vi "montecarlo bpsk.vi"() -> ()   [LabVIEW 2014]
uses:
  <vilib>/Analysis/NI_AALBase.lvlib
panel:
  out "XY Graph":cluster{"Y":dbl[], "Y":dbl[]}[](graph)
  out "Waveform Chart 2":dbl[][](graph)
  out "Waveform Chart":i32[](graph)
  in  "Numeric 5":i32
  in  "Numeric 4":i32
  in  "Numeric 3":i32
  in  "Numeric 2":i32
  in  "Numeric":i32
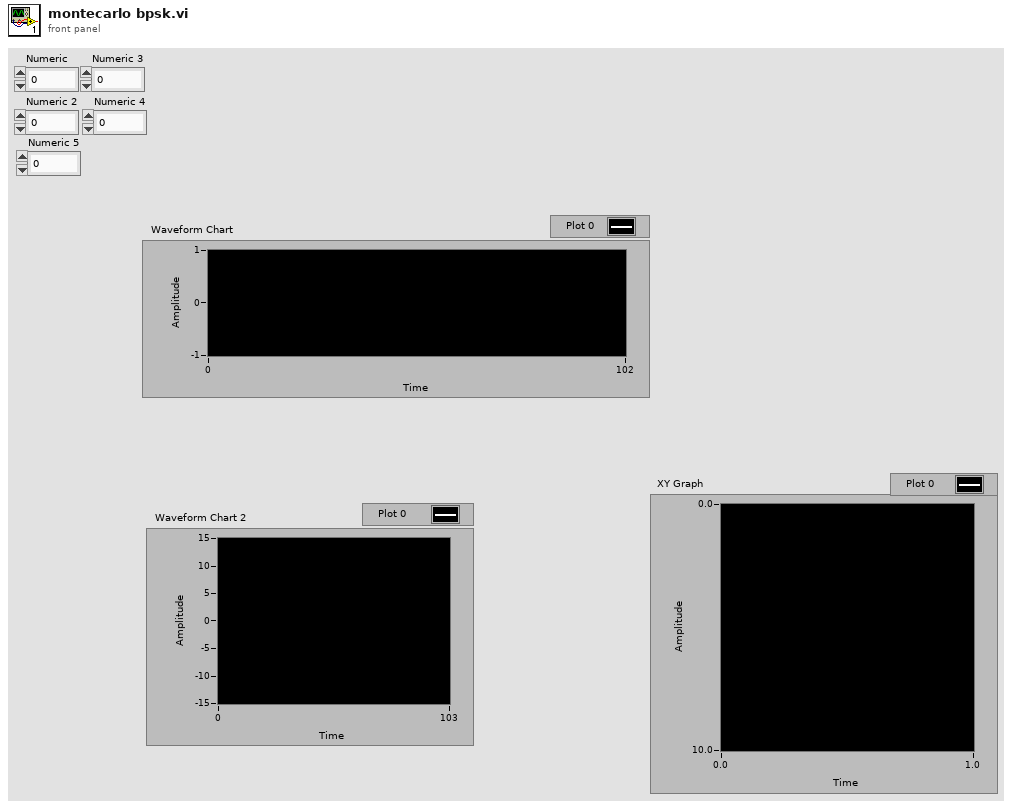
[diagram p1: front panel]
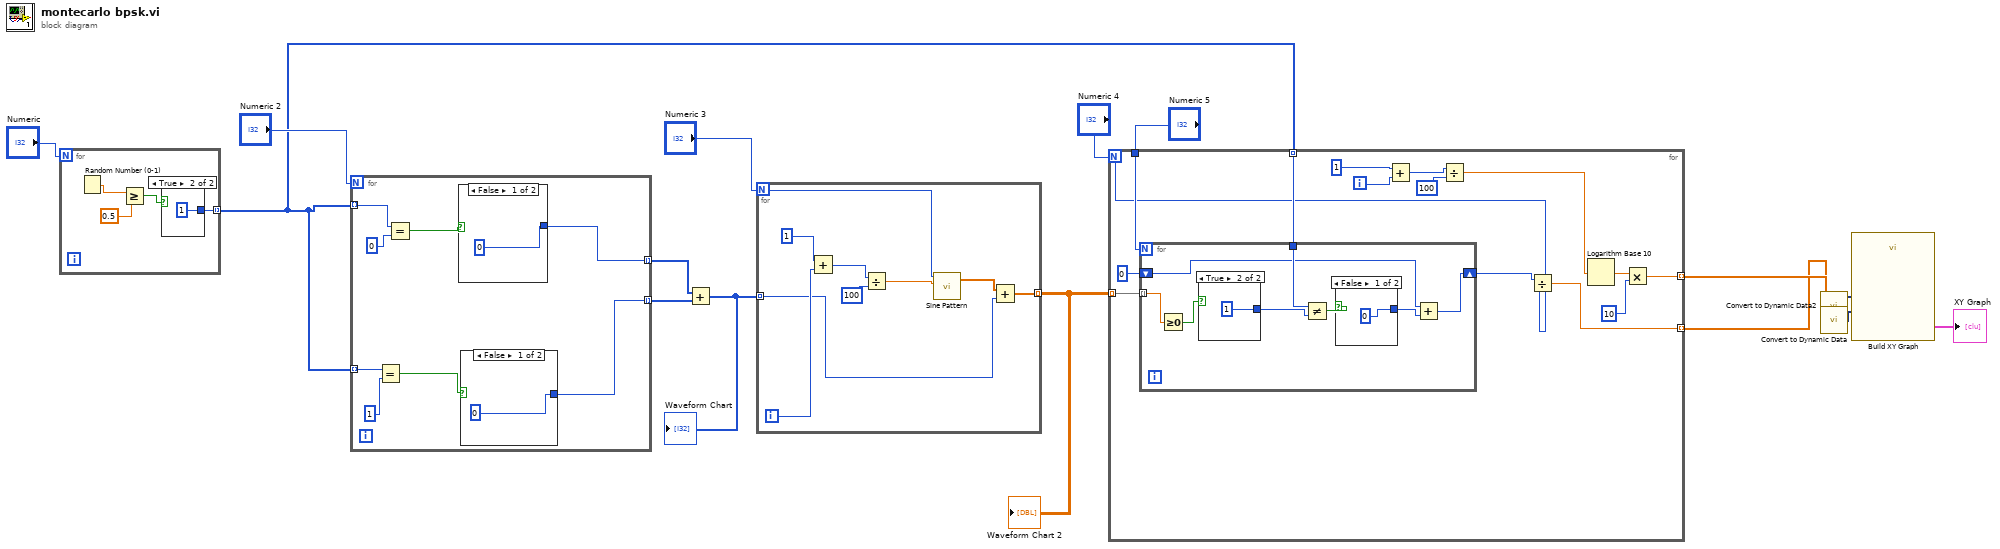
[diagram p0: block diagram]
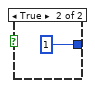
[diagram p2: hidden frame]
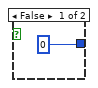
[diagram p3: hidden frame]
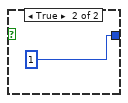
[diagram p4: hidden frame]
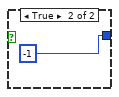
[diagram p5: hidden frame]
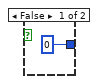
[diagram p6: hidden frame]
diagram:
  n1 = for {
    N: "Numeric" -> [_]
    tunnel: [w16] -> w8 mode=indexing
    n2 = Random Number (0-1)() -> (number: 0 to 1=w18:dbl)
    n3 = Greater Or Equal?(x=w18, y=0.5) -> (x >= y?=w17:bool)
    n4 = case shown="True" w17 {
      tunnel: [0 1] -> w16
      frame False {
      }
      frame True {
      }
    }
  }
  n5 = for {
    N: "Numeric 2" -> [_]
    tunnel: w8 -> [w28] mode=indexing
    tunnel: w8 -> [w26] mode=indexing
    tunnel: [w23] -> w13 mode=indexing
    tunnel: [w22] -> w12 mode=indexing
    n6 = Equal?(x=w26, y=1) -> (x = y?=w24:bool)
    n7 = Equal?(x=w28, y=0) -> (x = y?=w25:bool)
    n8 = case shown="False" w25 {
      tunnel: [0 -1] -> w23
      frame False {
      }
      frame True {
      }
    }
    n9 = case shown="False" w24 {
      tunnel: [0 1] -> w22
      frame False {
      }
      frame True {
      }
    }
  }
  n10 = Add(x=w13, y=w12) -> (x+y=w7:i32[])
  "Waveform Chart" <- w7
  n11 = for {
    N: "Numeric 3" -> [w37]
    tunnel: w7 -> [w36] mode=indexing
    tunnel: [w34] -> w6 mode=indexing
    i -> [w41]
    n12 = Add(x=1, y=w41) -> (x+y=w40:i32)
    n13 = Divide(x=w40, y=100) -> (x/y=w38:dbl)
    n14 = call <vilib>:"Sine Pattern.vi"("amplitude"=w38, "samples"=w37) -> ("Sinusoidal Pattern"=w35:dbl[])  [unwired: 2 in, 1 out]
    n15 = Add(x=w35, y=w36) -> (x+y=w34:dbl[])
  }
  "Waveform Chart 2" <- w6
  n16 = for {
    N: "Numeric 4" -> [w52]
    tunnel: "Numeric 5" -> [w57]
    tunnel: w6 -> [w56] mode=indexing
    tunnel: w8 -> [w55] mode=indexing
    tunnel: [w44] -> w4 mode=indexing
    tunnel: [w43] -> w2 mode=indexing
    i -> [w50]
    n17 = for {
      N: w57 -> [_]
      tunnel: w56 -> [w64] mode=indexing
      tunnel: w55 -> [w63]
      shift-right: [w60] -> w53
      shift-left: 0 -> [w58]
      n18 = Greater Or Equal To 0?(x=w64) -> (x >= 0?=w65:bool)
      n19 = case shown="True" w65 {
        tunnel: [0 1] -> w59
        frame False {
        }
        frame True {
        }
      }
      n20 = Not Equal?(x=w63, y=w59) -> (x != y?=w62:bool)
      n21 = case shown="False" w62 {
        tunnel: [0 1] -> w61
        frame False {
        }
        frame True {
        }
      }
      n22 = Add(x=w58, y=w61) -> (x+y=w60:i32)
    }
    n23 = Add(x=1, y=w50) -> (x+y=w49:i32)
    n24 = Divide(x=w49, y=100) -> (x/y=w47:dbl)
    n25 = Divide(x=w53, y=w52) -> (x/y=w43:dbl)
    n26 = Logarithm Base 10(1:w47) -> (0:w46:dbl)
    n27 = Multiply(x=w46, y=10) -> (x*y=w44:dbl)
  }
  n28 = call "Convert to Dynamic Data2"("Array"=w2) -> ("Dynamic Data Type"=w1:dynamicdata)  [unwired: 3 in]
  n29 = call "Convert to Dynamic Data"("Array"=w4) -> ("Dynamic Data Type"=w3:dynamicdata)  [unwired: 3 in]
  n30 = call "Build XY Graph"("Y Input"=w3, "X Input"=w1) -> ("XY Graph"=→"XY Graph":cluster{"X":dbl[], "Y":dbl[]}[])  [unwired: 8 in, 1 out]
